vi "CRYProject Run Control Global.vi"() -> ()   [LabVIEW 2013]
panel:
  out "ExitState":bool
  in  "Run Index Array":u32[](array[numeric])
  out "Run Stim steps only?":bool
  in  "Cont State":bool
  out "RunState":bool
  in  "Cancel fsw":bool
  in  "OK fsw":bool
  in  "Displayed":bool
  in  "Cont Seq":bool
  in  "Aborted":bool
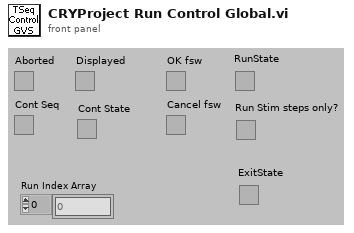
[diagram p1: front panel]
diagram:
